vi "Read Channel Array.vi"(8 "error in":errorcluster, 10 "channels":refnum<class "Channel.lvclass">[](array[class]), 11 "counter pwm input mode in":refnum<class "Counter PWM Input Mode.lvclass">) -> (0 "error out":errorcluster, 2 "channel settings":T1[](array[typedef]), 3 "counter pwm input mode out":refnum<class "Counter PWM Input Mode.lvclass">)   [LabVIEW 2017, in "Scan Engine Scripting.lvlib" / "Counter PWM Input Mode.lvclass"]
uses:
  Counter PWM Input Mode.lvclass
  Channel Classes/Channel/Channel.lvclass
  Controls/counter pwm input channel settings.ctl
  Channel Classes/PWM Input Channel/Measurement Type.ctl
  Counter PWM Input Mode.lvclass/Counter PWM Input Mode.ctl
  Channel Classes/PWM Input Channel/PWM Input Channel.lvclass
  Scan Engine Scripting.lvlib
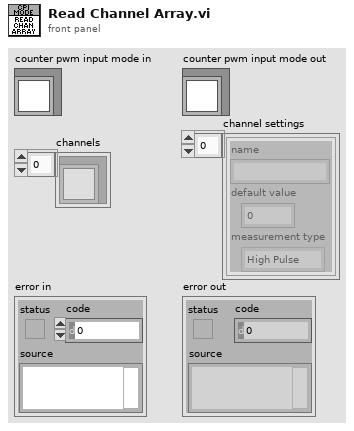
[diagram p1: front panel]
types:
  T1 = typedef "Scan Engine Scripting.lvlib/counter pwm input channel settings.ctl" = cluster{"name":string, "default value":dbl, "measurement type":T2}
  T2 = typedef "Scan Engine Scripting.lvlib/PWM Input Channel.lvclass/Measurement Type.ctl" = enum16{"High Pulse", "Low Pulse", "Most Recent"}
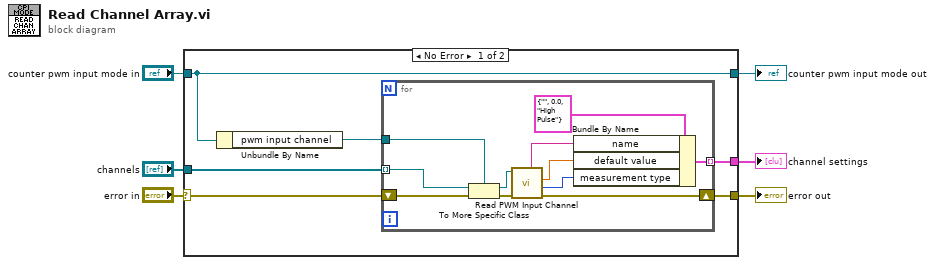
[diagram p0: block diagram]
diagram:
  n1 = case shown="No Error" "error in" {
    selector: "error in" -> [w11 w25]
    tunnel: [w10 w25] -> w5
    tunnel: [w8 w24] -> w3
    tunnel: "counter pwm input mode in" -> [w8 w24]
    tunnel: "channels" -> [w12 _]
    tunnel: [w9 _] -> w1
    frame No Error {
      n2 = Unbundle By Name(w8) -> ("pwm input channel"=w7:refnum<class "PWM Input Channel.lvclass">)
      n3 = for {
        tunnel: w12 -> [w20] mode=indexing
        tunnel: [w22] -> w9 mode=indexing
        shift-right: [w17] -> w10
        shift-left: w11 -> [w21]
        tunnel: w7 -> [w14]
        n4 = To More Specific Class(target class=w14, reference=w20, error in=w21) -> (specific class reference=w18:refnum<class "PWM Input Channel.lvclass">, error out=w19:errorcluster)
        n5 = call "Read PWM Input Channel.vi"("error in"=w19, "pwm input channel in"=w18) -> ("error out"=w17:errorcluster, "measurement type"=w13:T2, "default value"=w16:dbl, "name"=w15:string)  [unwired: 4 in, 2 out]
        n6 = Bundle By Name(cluster=T1 {"name"="", "default value"=0.0, "measurement type"=enum."High Pulse"} ("channel settings"), "name"=w15, "default value"=w16, "measurement type"=w13) -> (w22:T1)
      }
    }
    frame Error {
    }
  }
  "error out" <- w5
  "counter pwm input mode out" <- w3
  "channel settings" <- w1
